vi "User@DisableControl__Parameter.vi"(1 "ParamterIn":string) -> (0 "ParamterOut":string)   [LabVIEW 2020]
panel:
  in  "Parameters":string(combo)
  in  "UserPanelControl":string(combo)
  in  "Confirm":bool
  # "User@DisableControl $UserPanelControlName(,$Parameter)"
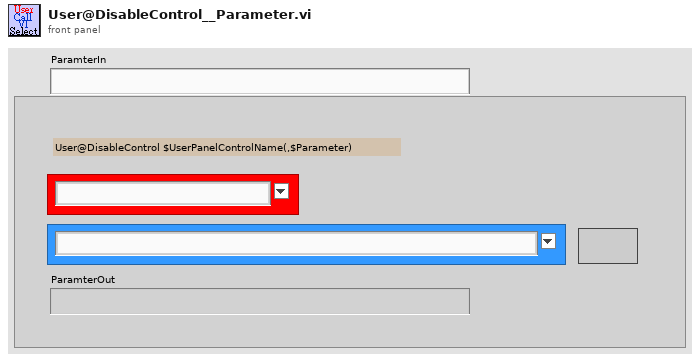
[diagram p1: front panel]
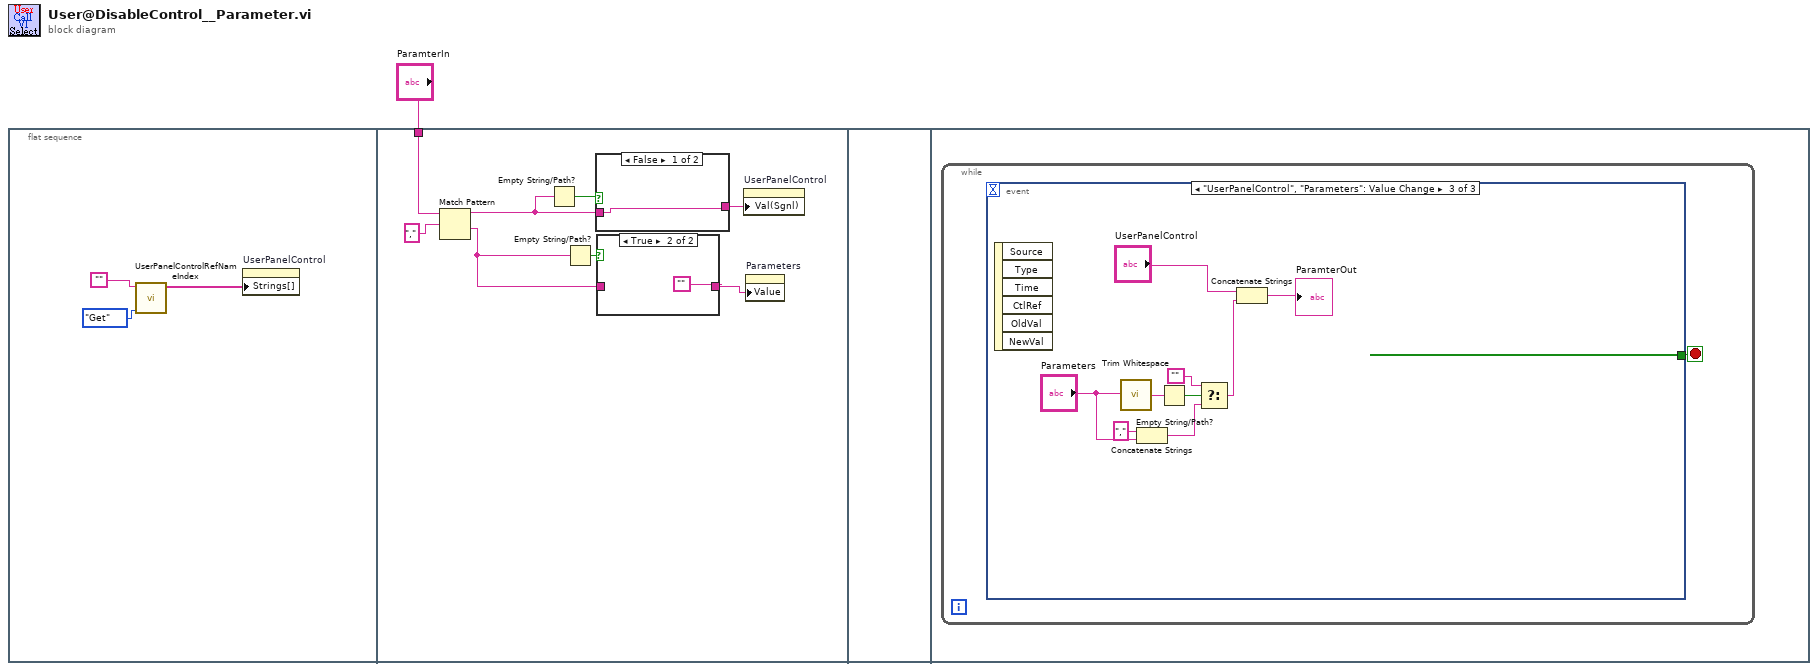
[diagram p0: block diagram]
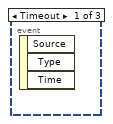
[diagram p4: hidden frame]
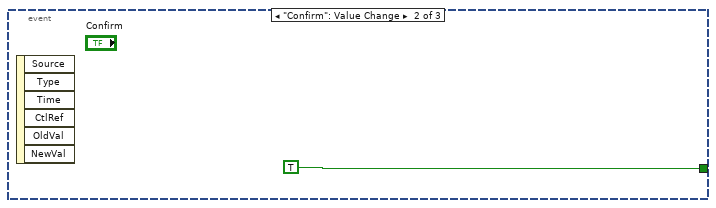
[diagram p5: hidden frame]
diagram:
  n1 = flat-sequence {
    tunnel: "ParamterIn" -> [w10]
    frame #0 {
      n2 = call "UserPanelControlRefNameIndex.vi"("OP"=enum16{"Get", "Update", "Init"}."Get", "ControlName"="") -> ("ControlNameS"=w2:string[])  [unwired: 6 in, 3 out]
      n3 = property on="UserPanelControl" class="CmbBox"("Strings[]"=w2) -> ()  [unwired: 2 in, 2 out]
    }
    frame #1 {
      n4 = Match Pattern(string=w10, regular expression=",") -> (before substring=w8:string, after substring=w7:string)  [unwired: 1 in, 2 out]
      n5 = Empty String/Path?(string/path=w8) -> (empty?=w12:bool)
      n6 = Empty String/Path?(string/path=w7) -> (empty?=w11:bool)
      n7 = case shown="False" w12 {
        tunnel: w8 -> [w15 w16]
        tunnel: [w15 w16] -> w5
        frame False {
        }
        frame True {
        }
      }
      n8 = case shown="True" w11 {
        tunnel: [w13 ""] -> w6
        tunnel: w7 -> [w13 _]
        frame False {
        }
        frame True {
        }
      }
      n9 = property on="UserPanelControl" class="CmbBox"("Val(Sgnl)"=w5) -> ()  [unwired: 2 in, 2 out]
      n10 = property on="Parameters" class="CmbBox"("Value"=w6) -> ()  [unwired: 2 in, 2 out]
    }
    frame #2 {
    }
    frame #3 {
      n11 = while {
        stop <- w17 stop-if-true
        n12 = event shown="[2] \"UserPanelControl\", \"Parameters\": Value Change" {
          selector: _ -> [_ _ _]
          dyn-events: _ -> [_ _ _]
          timeout: _ -> [_ _ _]
          tunnel: [_ TRUE _] -> w17
          event Timeout {
            n13 = event-data() -> ()  [unwired: 1 in, 3 out]
          }
          event "Confirm": Value Change {
            n14 = event-data() -> ()  [unwired: 1 in, 6 out]
          }
          event "UserPanelControl", "Parameters": Value Change {
            n15 = event-data() -> ()  [unwired: 1 in, 6 out]
            n16 = call <vilib>:"Trim Whitespace.vi"("string"="Parameters") -> ("trimmed string"=w23:string)  [unwired: 1 in]
            n17 = Concatenate Strings("," ("string"), "Parameters") -> (w22:string)
            n18 = Empty String/Path?(string/path=w23) -> (empty?=w24:bool)
            n19 = Select(t="", s=w24, f=w22) -> (s? t:f=w19:string)
            n20 = Concatenate Strings("UserPanelControl", w19) -> (→"ParamterOut":string)
          }
        }
      }
    }
  }
